vi "STL-ArrayToCanvas.vi"(9 "Scale":i32=50, 10 "STL array":dbl[][](array[numeric]), 11 "Picture In":picture) -> (3 "Picture Out":picture)   [LabVIEW 2019]
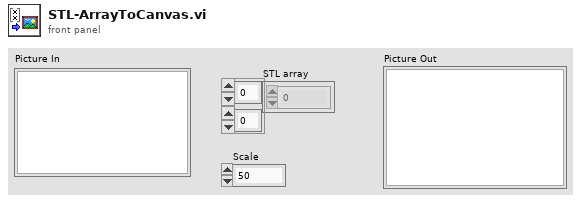
[diagram p1: front panel]
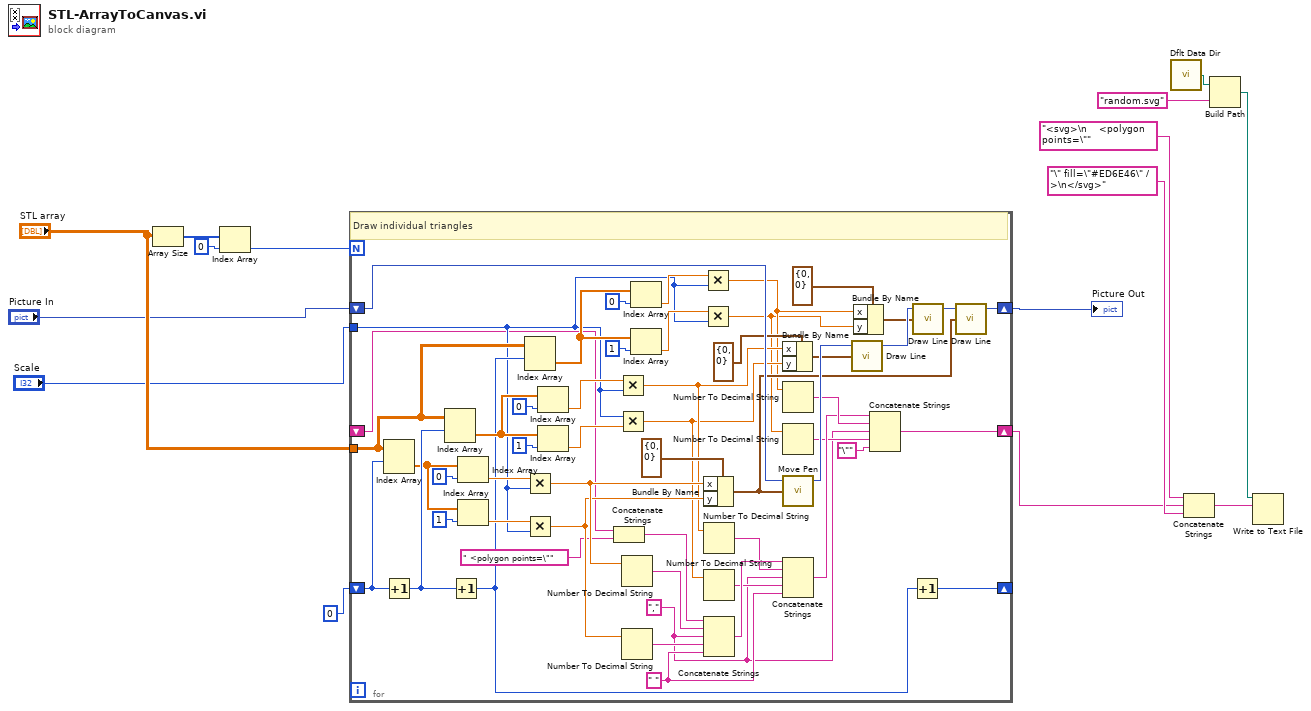
[diagram p0: block diagram]
diagram:
  n1 = Array Size(array="STL array") -> (size(s)=w13:i32[])
  n2 = Index Array(array=w13, index=0) -> (element=w15:i32)
  n3 = for {
    N: w15 -> [_]
    tunnel: "STL array" -> [w67]
    shift-right: [w40] -> _
    shift-left: 0 -> [w43]
    shift-right: [w38] -> w10
    shift-left: "Picture In" -> [w66]
    tunnel: "Scale" -> [w44]
    shift-right: [w36] -> w1
    shift-left: _ -> [w19]
    w26 = " " ("string")
    w16 = "," ("string")
    # "Draw individual triangles"
    n4 = Index Array(array=w67, index (row)=w43) -> (element=w57:dbl[])  [unwired: 1 in]
    n5 = Increment(x=w43) -> (x+1=w68:i32)
    n6 = Index Array(array=w67, index (row)=w68) -> (element=w56:dbl[])  [unwired: 1 in]
    n7 = Increment(x=w68) -> (x+1=w45:i32)
    n8 = Index Array(array=w57, index=0) -> (element=w51:dbl)
    n9 = Index Array(array=w57, index=1) -> (element=w50:dbl)
    n10 = Index Array(array=w67, index (row)=w45) -> (element=w55:dbl[])  [unwired: 1 in]
    n11 = Multiply(x=w51, y=w44) -> (x*y=w35:dbl)
    n12 = Multiply(x=w50, y=w44) -> (x*y=w33:dbl)
    n13 = Index Array(array=w56, index=0) -> (element=w49:dbl)
    n14 = Index Array(array=w56, index=1) -> (element=w48:dbl)
    n15 = Concatenate Strings(w19, " <polygon points=\"" ("string")) -> (w17:string)
    n16 = Multiply(x=w49, y=w44) -> (x*y=w30:dbl)
    n17 = Multiply(x=w44, y=w48) -> (x*y=w28:dbl)
    n18 = Number To Decimal String(number=w35) -> (decimal integer string=w34:string)  [unwired: 1 in]
    n19 = Number To Decimal String(number=w33) -> (decimal integer string=w32:string)  [unwired: 1 in]
    n20 = Index Array(array=w55, index=0) -> (element=w47:dbl)
    n21 = Index Array(array=w55, index=1) -> (element=w46:dbl)
    n22 = Multiply(x=w47, y=w44) -> (x*y=w25:dbl)
    n23 = Multiply(x=w46, y=w44) -> (x*y=w21:dbl)
    n24 = Bundle By Name(cluster=cluster{"x":i16, "y":i16} {"x"=0, "y"=0} ("end point"), "x"=w35, "y"=w33) -> (w37:cluster{"x":i16, "y":i16})
    n25 = Number To Decimal String(number=w30) -> (decimal integer string=w29:string)  [unwired: 1 in]
    n26 = Number To Decimal String(number=w28) -> (decimal integer string=w27:string)  [unwired: 1 in]
    n27 = Concatenate Strings(w17, w34, w16, w32, w26) -> (w31:string)
    n28 = Bundle By Name(cluster=cluster{"x":i16, "y":i16} {"x"=0, "y"=0} ("end point"), "x"=w30, "y"=w28) -> (w41:cluster{"x":i16, "y":i16})
    n29 = Number To Decimal String(number=w25) -> (decimal integer string=w24:string)  [unwired: 1 in]
    n30 = Number To Decimal String(number=w21) -> (decimal integer string=w22:string)  [unwired: 1 in]
    n31 = call <vilib>:"Move Pen.vi"("new position"=w37, "picture"=w66) -> ("new picture"=w65:picture)  [unwired: 3 in]
    n32 = Concatenate Strings(w31, w29, w16, w27, w26) -> (w23:string)
    n33 = call <vilib>:"Draw Line.vi"("picture"=w65, "end point"=w41) -> ("new picture"=w64:picture)  [unwired: 7 in]
    n34 = Bundle By Name(cluster=cluster{"x":i16, "y":i16} {"x"=0, "y"=0} ("end point"), "x"=w25, "y"=w21) -> (w42:cluster{"x":i16, "y":i16})
    n35 = Concatenate Strings(w23, w24, w16, w22, "\"" ("string")) -> (w36:string)
    n36 = Increment(x=w45) -> (x+1=w40:i32)
    n37 = call <vilib>:"Draw Line.vi"("picture"=w64, "end point"=w42) -> ("new picture"=w39:picture)  [unwired: 7 in]
    n38 = call <vilib>:"Draw Line.vi"("picture"=w39, "end point"=w37) -> ("new picture"=w38:picture)  [unwired: 7 in]
  }
  "Picture Out" <- w10
  n39 = call <vilib>:"Dflt Data Dir.vi"() -> ("App:Default Data Directory"=w7:path)
  n40 = Concatenate Strings("<svg>\n    <polygon points=\"" ("string"), w1, "\" fill=\"#ED6E46\" />\n</svg>") -> (w2:string)
  n41 = Build Path(base path=w7, name or relative path="random.svg") -> (appended path=w5:path)
  n42 = Write to Text File(file (use dialog)=w5, text=w2) -> ()  [unwired: 2 in, 3 out]
